vi "000_Bool True.vi"(10 "Value":bool, 11 "Bool String":string) -> (1 "Anti":string, 2 "String Out":string, 3 "True":bool)   [LabVIEW 2020]
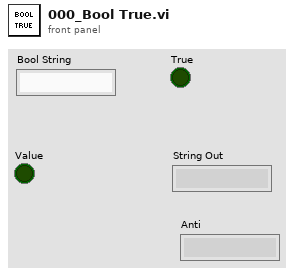
[diagram p1: front panel]
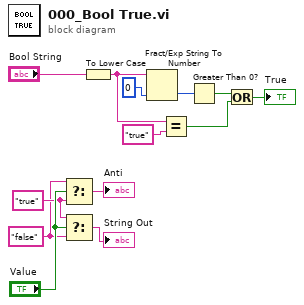
[diagram p0: block diagram]
diagram:
  w2 = "false" ("f")
  w3 = "true" ("y")
  n1 = Select(t=w2, s="Value", f=w3) -> (s? t:f=→"Anti":string)
  n2 = Select(t=w3, s="Value", f=w2) -> (s? t:f=→"String Out":string)
  n3 = To Lower Case(string="Bool String") -> (all lower case string=w5:string)
  n4 = Fract/Exp String To Number(string=w5, default (0 dbl)=0 ("默认(0 DBL)")) -> (number=w11:i32)  [unwired: 2 in, 1 out]
  n5 = Equal?(x=w5, y="true") -> (x = y?=w9:bool)
  n6 = Greater Than 0?(x=w11) -> (x > 0?=w10:bool)
  n7 = Or(x=w10, y=w9) -> (x .or. y?=→"True":bool)
